vi "Convert_allValues.vi"(4 "Accel (MPU6050) Offset":dbl, 6 "Load (Futek) Offset":dbl, 7 "Grip (Omega) Value":dbl, 8 "Grip (Omega) Offset":dbl, 10 "Accel (MPU6050) Value":dbl, 11 "Load (Futek) Value":dbl) -> (0 "Dynamic Load Force":dbl, 1 "Static Load Force":dbl, 2 "Grip Force":dbl)   [LabVIEW 2020]
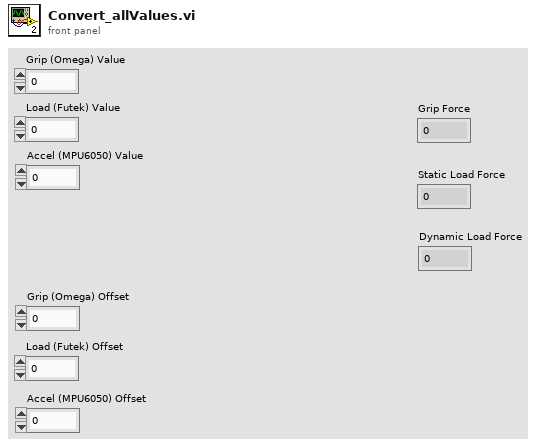
[diagram p1: front panel]
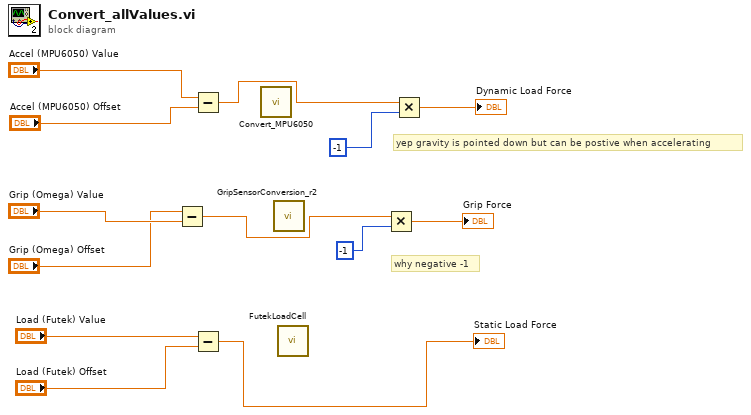
[diagram p0: block diagram]
diagram:
  # "yep gravity is pointed down but can be postive when accelerating"
  # "why negative -1"
  n1 = Subtract(x="Grip (Omega) Offset", y="Grip (Omega) Value") -> (x-y=w2:dbl)
  n2 = Subtract(x="Accel (MPU6050) Value", y="Accel (MPU6050) Offset") -> (x-y=w3:dbl)
  n3 = Subtract(x="Load (Futek) Value", y="Load (Futek) Offset") -> (x-y=→"Static Load Force":dbl)
  n4 = call "Convert_MPU6050.vi"() -> ()  [unwired: 1 in, 1 out]
  n5 = call "GripSensorConversion_r2.vi"() -> ()  [unwired: 1 in, 1 out]
  n6 = call "FutekLoadCell.vi"() -> ()  [unwired: 1 in, 1 out]
  n7 = Multiply(x=w2, y=-1) -> (x*y=→"Grip Force":dbl)
  n8 = Multiply(x=w3, y=-1) -> (x*y=→"Dynamic Load Force":dbl)
